vi "Begin.vi"() -> (0 "error out":errorcluster, 1 "CameraDevRef":T1)   [LabVIEW 2011]
doc: "Called before other user functions, this VI is expected to open initial I/O refnums, load in file data, and do all program initialization. Notice that the <B>error out</B> terminal is simply used for data flow. Wiring it to other structures or subVIs ensures that this VI runs first."
uses:
  Robot Global Data.vi
  <vilib>/Rock Robotics/WPI/MotorControl/WPI_MotorControlOpen Victor.vi
  <vilib>/Rock Robotics/SystemInterfaces/DIO/FPGA_DIOPWMChannel.ctl
  <vilib>/Rock Robotics/WPI/Joystick/WPI_JoystickDeviceEnum.ctl
  <vilib>/Rock Robotics/SystemInterfaces/DIO/FPGA_DIORelayChannel.ctl
  <vilib>/Rock Robotics/WPI/Relay/WPI_RelayDirection.ctl
  <vilib>/Rock Robotics/SystemInterfaces/Typedef/FPGA_TypedefDigitalModule.ctl
  <vilib>/Rock Robotics/SystemInterfaces/AI/FPGA_AIChannel.ctl
  <vilib>/Rock Robotics/WPI/Counter/WPI_CounterDigitalInputToDigitalSource.vi
  <vilib>/Rock Robotics/SystemInterfaces/DIO/FPGA_DIOChannel.ctl
  <vilib>/Rock Robotics/WPI/Encoder/WPI_EncoderType.ctl
  <vilib>/Rock Robotics/SystemInterfaces/AI/FPGA_AIGyroChannel.ctl
  <vilib>/Rock Robotics/WPI/MotorControl/WPI_MotorControlOpen Jaguar.vi
  <vilib>/Utility/file.llb/Read From Spreadsheet File (DBL).vi
  <vilib>/Rock Robotics/WPI/Camera/WPI_CameraDevRef.ctl
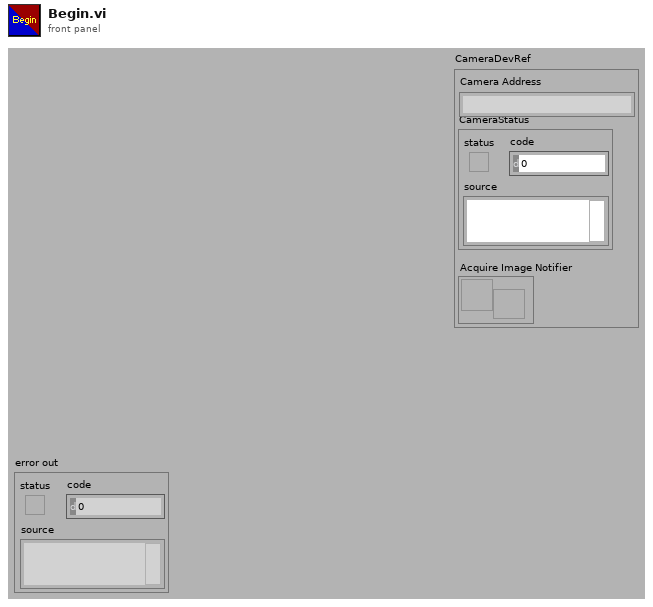
[diagram p1: front panel]
types:
  T1 = typedef "WPI_CameraDevRef.ctl" = cluster{"Camera Address":string, "CameraStatus":errorcluster, "Acquire Image Notifier":refnum<notifier>}
  T2 = typedef "FPGA_TypedefDigitalModule.ctl" = enum16{"Digital Module 1", "Digital Module 2"}
  T3 = typedef "FPGA_DIOPWMChannel.ctl" = enum8{"PWM 1", "PWM 2", "PWM 3", "PWM 4", "PWM 5", "PWM 6", "PWM 7", "PWM 8", "PWM 9", "PWM 10", "Invalid"}
  T4 = typedef "FPGA_AIGyroChannel.ctl" = enum8{"AI 1", "AI 2", "Invalid"}
  T5 = typedef "WPI_EncoderType.ctl" = enum16{"1x", "2x", "4x"}
  T6 = typedef "FPGA_DIOChannel.ctl" = enum8{"DIO 1", "DIO 2", "DIO 3", "DIO 4", "DIO 5", "DIO 6", "DIO 7", "DIO 8", "DIO 9", "DIO 10", "DIO 11", "DIO 12", "DIO 13", "DIO 14", "Invalid"}
  T7 = typedef "FPGA_AIChannel.ctl" = enum8{"AI 1", "AI 2", "AI 3", "AI 4", "AI 5", "AI 6", "AI 7", "AI 8", "Invalid"}
  T8 = typedef "FPGA_DIORelayChannel.ctl" = enum8{"Relay 1", "Relay 2", "Relay 3", "Relay 4", "Relay 5", "Relay 6", "Relay 7", "Relay 8", "Invalid"}
  T9 = typedef "WPI_RelayDirection.ctl" = enum16{"Both directions", "Forward only", "Reverse only"}
  T10 = typedef "WPI_JoystickDeviceEnum.ctl" = enum16{"USB 1", "USB 2", "USB 3", "USB 4", "Kinect 1", "Kinect 2"}
  T11 = typedef "WPI_CameraImageSize.ctl" = enum16{"640x480", "320x240", "160x120"}
  T12 = cluster{"fps":i32, "compression":i32, "Image Size":T11}
  T13 = typedef "WPI_I2CDevRef.ctl" = cluster{"DevStatus":errorcluster, "Digital Module":T2, "Device Address":u8}
  T14 = typedef "WPI_DigitalInputDevRef.ctl" = cluster{"DevStatus":errorcluster, "DIO Channel":T6, "Digital Module":T2}
  T15 = typedef "FPGA_CounterEncoderSourceConvertionLVSourceType.ctl" = cluster{"DevStatus":errorcluster, "AnalogTriggerMode?":bool, "DigitalMode":cluster{"Digital Module":T2, "DIO Channel":T16}, "AnalogTriggerMode":cluster{"AnalogTriggerIndex":T17, "OutputType":T18}}
  T16 = typedef "FPGA_DIODigitalSourceChannel.ctl" = enum8{"DIO 1", "DIO 2", "DIO 3", "DIO 4", "DIO 5", "DIO 6", "DIO 7", "DIO 8", "DIO 9", "DIO 10", "DIO 11", "DIO 12", "DIO 13", "DIO 14", "Disabled"}
  T17 = typedef "FPGA_AnalogTriggerIndex.ctl" = enum8{"Trig 0", "Trig 1", "Trig 2", "Trig 3", "Trig 4", "Trig 5", "Trig 6", "Trig 7", "Invalid"}
  T18 = typedef "FPGA_AnalogTriggerOutType.ctl" = enum16{"InWindow", "TriggerState", "Rising", "Falling"}
  T19 = typedef "WPI_MotorControlDeviceRef.ctl" = cluster{"DeviceStatus":errorcluster, "Type":enum16{"PWM", "CAN"}, "PWM":cluster{"Digital Module":T2, "PWM Channel":T3, "DeadBand":T20}, "CAN":cluster{"Device Number":u8, "Control Mode":T21, "Semaphore":T22, "Max Vout":dbl}, "Invert":bool, "TransformRef":T23, "InvTransformRef":T23}
  T20 = typedef "WPI_PWMDeadband.ctl" = cluster{"Name":string, "maxPositivePwm":i32, "minPositivePwm":i32, "centerPwm":i32, "maxNegativePwm":i32, "minNegativePwm":i32, "angularRange":u16}
  T21 = typedef "WPI_CANJaguar_ControlMode.ctl" = enum8{"Percent VBus", "Current", "Speed", "Position", "Voltage"}
  T22 = typedef "Semaphore RefNum" = refnum<k1>
  T23 = typedef "WPI_PWMTransform_ConPane.ctl" = refnum<vi>
  T24 = typedef "WPI_EncoderDevRef.ctl" = cluster{"DevStatus":errorcluster, "EncoderIndex":T25, "CounterIndex":T26, "DistancePerCount":dbl, "Decoding Type":T5}
  T25 = typedef "FPGA_EncoderIdx.ctl" = enum8{"Enc 0", "Enc 1", "Enc 2", "Enc 3", "Invalid"}
  T26 = typedef "FPGA_CounterCtrSystemIndex.ctl" = enum8{"Ctr 0", "Ctr 1", "Ctr 2", "Ctr 3", "Ctr 4", "Ctr 5", "Ctr 6", "Ctr 7", "Invalid"}
  T27 = typedef "WPI_CameraWhite Balance Values.ctl" = enum16{"Auto", "Fixed indoor", "Fixed outdoor 1", "Fixed outdoor 2", "Fixed fluorescent 1", "Fixed fluorescent 2", "Hold current"}
  T28 = typedef "WPI_CameraExposure Values.ctl" = enum16{"Auto", "Flicker-free 50 Hz", "Flicker-free 60 Hz", "Hold current"}
  T29 = typedef "WPI_ServoDeviceRef.ctl" = cluster{"DeviceStatus":errorcluster, "Digital Module":T2, "PWM Channel":T3, "DeadBand":T20}
  T30 = typedef "WPI_AnalogChannelDevRef.ctl" = cluster{"DevStatus":errorcluster, "Analog Module":T31, "Analog Channel":T7}
  T31 = typedef "FPGA_TypedefAnalogModule.ctl" = enum16{"Analog Module 1", "Analog Module 2"}
  T32 = typedef "WPI_JoystickDevRef.ctl" = cluster{"Device":T10}
  T33 = typedef "WPI_GyroDevRef.ctl" = cluster{"DevStatus":errorcluster, "Analog Module":T31, "Analog Channel":T7, "Offset":dbl, "Gain (VoltsPerDegree/Second)":dbl}
  T34 = typedef "WPI_RelayDevRef.ctl" = cluster{"DevStatus":errorcluster, "Relay Channel":T8, "Digital Module":T2, "Relay Direction":T9}
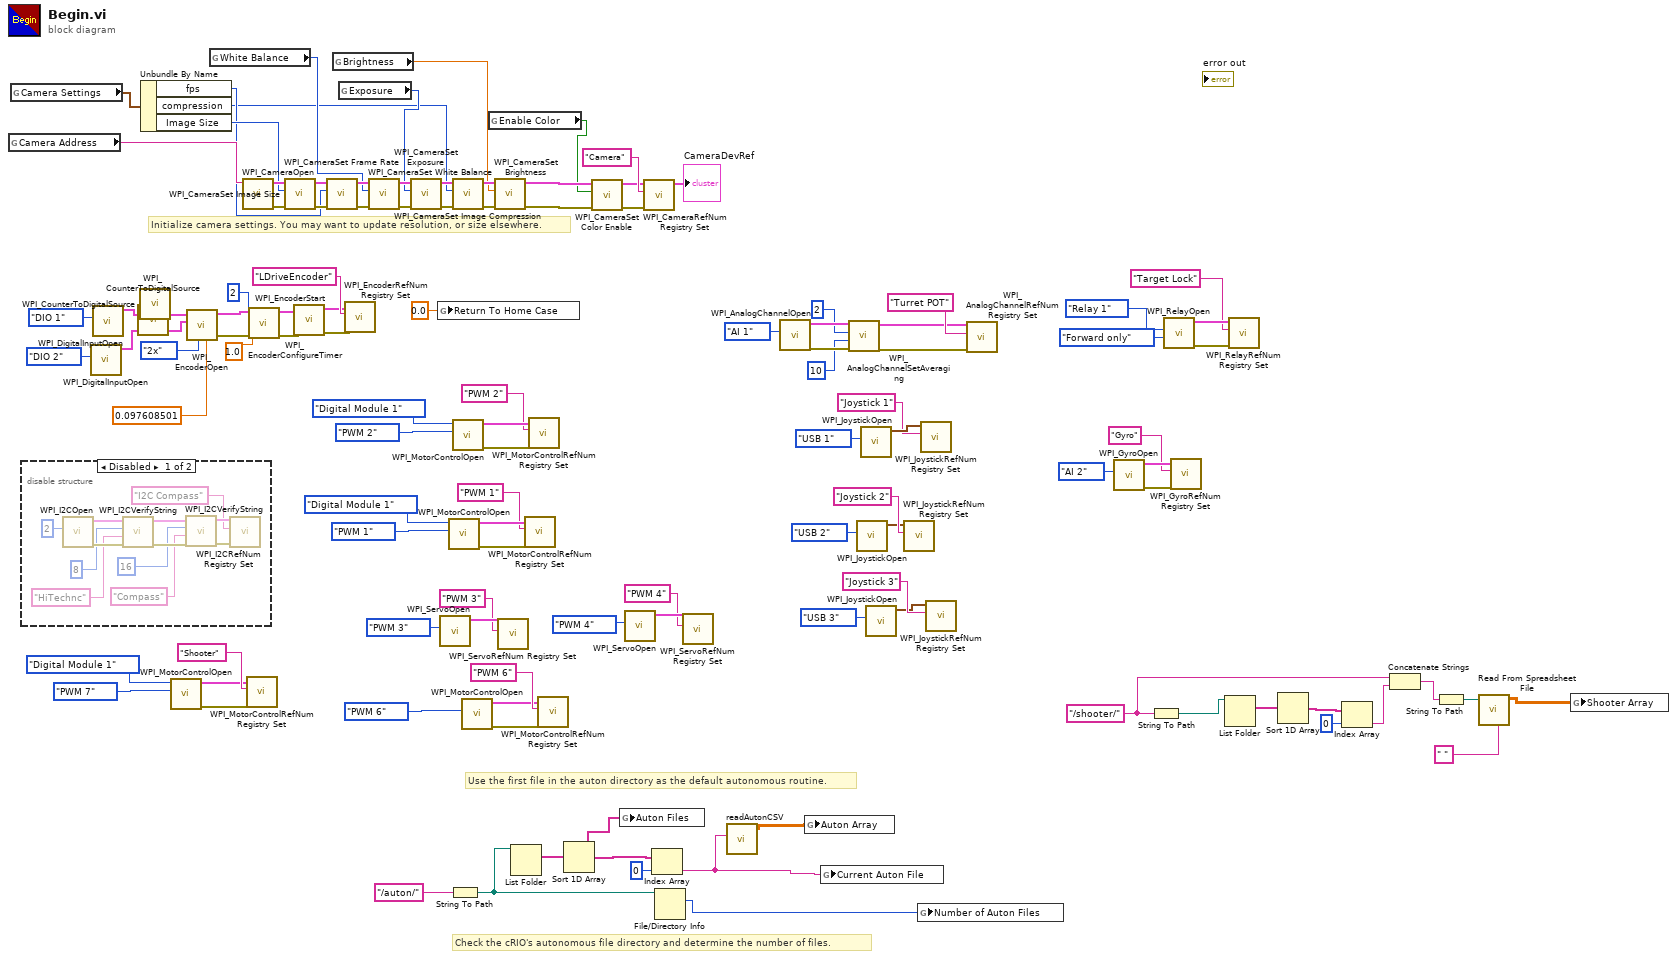
[diagram p0: block diagram]
diagram:
  w11 = "/shooter/" ("string")
  # "Check the cRIO's autonomous file directory and determine the number of files."
  # "Use the first file in the auton directory as the default autonomous routine."
  # "Initialize camera settings. You may want to update resolution, or size elsewhere."
  n1 = global read "Robot Global Data.vi" "Camera Address"() -> (w101:string)
  n2 = global read "Robot Global Data.vi" "Camera Settings"() -> (w73:T12)
  n3 = disable-structure shown="Disabled" {
    frame Disabled {
      n4 = call <vilib>:"WPI_I2COpen.vi"("Device Address"=u8 2) -> ("error out"=w126:errorcluster, "I2CDevRef"=w125:T13)  [unwired: 9 in]
      n5 = call <vilib>:"WPI_I2CVerifyString.vi"("error in (no error)"=w126, "Expected"="HiTechnc", "Register Address"=u8 8, "I2CDevRef"=w125) -> ("error out"=w124:errorcluster, "I2CDevRef"=w123:T13)  [unwired: 6 in]
      n6 = call <vilib>:"WPI_I2CVerifyString.vi"("error in (no error)"=w124, "Expected"="Compass", "Register Address"=u8 16, "I2CDevRef"=w123) -> ("error out"=w122:errorcluster, "I2CDevRef"=w121:T13)  [unwired: 6 in]
      n7 = call <vilib>:"WPI_I2CRefNum Registry Set.vi"("error in (no error)"=w122, "refnum name"="I2C Compass", "I2CDevRef"=w121) -> ()  [unwired: 7 in, 2 out]
    }
    frame Enabled {
    }
  }
  n8 = call <vilib>:"WPI_DigitalInputOpen.vi"("DIO Channel"=FPGA_DIOChannel."DIO 2") -> ("DigitalInputDevRef"=w38:T14)  [unwired: 9 in, 1 out]
  n9 = call <vilib>:"WPI_DigitalInputOpen.vi"("DIO Channel"=FPGA_DIOChannel."DIO 1") -> ("DigitalInputDevRef"=w41:T14)  [unwired: 9 in, 1 out]
  n10 = call-poly <vilib>:"WPI_CounterToDigitalSource.vi"("DigitalInputDevRef"=w38) -> ("Digital Source"=w37:T15)  [unwired: 6 in]
  n11 = call-poly <vilib>:"WPI_CounterToDigitalSource.vi"("DigitalInputDevRef"=w41) -> ("Digital Source"=w42:T15)  [unwired: 6 in]
  n12 = Unbundle By Name(w73) -> ("fps"=w71:i32, "compression"=w68:i32, "Image Size"=w72:T11)
  n13 = call-poly <vilib>:"WPI_MotorControlOpen.vi"("PWM Channel"=FPGA_DIOPWMChannel."PWM 7", "Digital Module (Module 1)"=FPGA_TypedefDigitalModule."Digital Module 1") -> ("error out"=w20:errorcluster, "MotorControlDeviceRef"=w18:T19)  [unwired: 8 in]
  n14 = call <vilib>:"WPI_EncoderOpen.vi"("DistancePerCount"=0.097608501, "Decoding Type"=WPI_EncoderType."2x", "BSource"=w37, "ASource"=w42) -> ("error out"=w33:errorcluster, "EncoderDevRef"=w32:T24)  [unwired: 6 in]
  n15 = global read "Robot Global Data.vi" "White Balance"() -> (w70:T27)
  n16 = call <vilib>:"WPI_CameraOpen.vi"("Camera Address"=w101) -> ("error out"=w107:errorcluster, "CameraDevRef"=w108:T1)  [unwired: 1 in, 8 out]
  n17 = call <vilib>:"WPI_MotorControlRefNum Registry Set.vi"("error in (no error)"=w20, "refnum name"="Shooter", "MotorControlDevRef"=w18) -> ()  [unwired: 7 in, 2 out]
  n18 = call <vilib>:"WPI_EncoderConfigureTimer.vi"("error in (no error)"=w33, "Number Samples to Average"=u8 2, "Minimum Rate"=1.0, "EncoderDevRef"=w32) -> ("error out"=w28:errorcluster, "EncoderDevRef"=w29:T24)  [unwired: 6 in]
  n19 = call <vilib>:"WPI_CameraSet Image Size.vi"("error in (no error)"=w107, "Image Size"=w72, "CameraDevRef"=w108) -> ("error out"=w106:errorcluster, "CameraDevRef Out"=w109:T1)  [unwired: 7 out]
  n20 = call <vilib>:"WPI_EncoderStart.vi"("error in (no error)"=w28, "EncoderDevRef"=w29) -> ("error out"=w26:errorcluster, "EncoderDevRef"=w27:T24)  [unwired: 8 in]
  n21 = call <vilib>:"WPI_CameraSet Frame Rate.vi"("error in (no error)"=w106, "Frame Rate (fps)"=w71, "CameraDevRef"=w109) -> ("error out"=w105:errorcluster, "CameraDevRef Out"=w111:T1)  [unwired: 7 out]
  n22 = global read "Robot Global Data.vi" "Brightness"() -> (w67:dbl)
  n23 = global read "Robot Global Data.vi" "Exposure"() -> (w69:T28)
  n24 = call <vilib>:"WPI_EncoderRefNum Registry Set.vi"("error in (no error)"=w26, "refnum name"="LDriveEncoder", "EncoderDevRef"=w27) -> ()  [unwired: 7 in, 2 out]
  n25 = call <vilib>:"WPI_CameraSet White Balance.vi"("error in (no error)"=w105, "White Balance"=w70, "CameraDevRef"=w111) -> ("error out"=w104:errorcluster, "CameraDevRef Out"=w110:T1)  [unwired: 7 out]
  n26 = call <vilib>:"WPI_CameraSet Exposure.vi"("error in (no error)"=w104, "Exposure"=w69, "CameraDevRef"=w110) -> ("error out"=w103:errorcluster, "CameraDevRef Out"=w113:T1)  [unwired: 7 out]
  n27 = global write "Robot Global Data.vi" "Return To Home Case"(0.0 ("Return To Home Case")) -> ()
  n28 = call <vilib>:"WPI_ServoOpen.vi"("PWM Channel"=FPGA_DIOPWMChannel."PWM 3") -> ("ServoDeviceRef"=w87:T29)  [unwired: 9 in, 1 out]
  n29 = call-poly <vilib>:"WPI_MotorControlOpen.vi"("PWM Channel"=FPGA_DIOPWMChannel."PWM 1", "Digital Module (Module 1)"=FPGA_TypedefDigitalModule."Digital Module 1") -> ("error out"=w93:errorcluster, "MotorControlDeviceRef"=w96:T19)  [unwired: 8 in]
  n30 = String To Path(string="/auton/") -> (path=w49:path)
  n31 = call <vilib>:"WPI_CameraSet Image Compression.vi"("error in (no error)"=w103, "Compression"=w68, "CameraDevRef"=w113) -> ("error out"=w102:errorcluster, "CameraDevRef Out"=w112:T1)  [unwired: 7 out]
  n32 = call-poly <vilib>:"WPI_MotorControlOpen.vi"("PWM Channel"=FPGA_DIOPWMChannel."PWM 2", "Digital Module (Module 1)"=FPGA_TypedefDigitalModule."Digital Module 1") -> ("error out"=w94:errorcluster, "MotorControlDeviceRef"=w99:T19)  [unwired: 8 in]
  n33 = call-poly <vilib>:"WPI_MotorControlOpen.vi"("PWM Channel"=FPGA_DIOPWMChannel."PWM 6") -> ("error out"=w82:errorcluster, "MotorControlDeviceRef"=w80:T19)  [unwired: 9 in]
  n34 = global read "Robot Global Data.vi" "Enable Color"() -> (w62:bool)
  n35 = call <vilib>:"WPI_CameraSet Brightness.vi"("error in (no error)"=w102, "Brightness"=w67, "CameraDevRef"=w112) -> ("error out"=w65:errorcluster, "CameraDevRef Out"=w66:T1)  [unwired: 7 out]
  n36 = call <vilib>:"WPI_ServoRefNum Registry Set.vi"("refnum name"="PWM 3", "ServoDeviceRef"=w87) -> ()  [unwired: 8 in, 2 out]
  n37 = List Folder(path=w49) -> (filenames=w48:string[])  [unwired: 1 in, 5 out]
  n38 = call <vilib>:"WPI_MotorControlRefNum Registry Set.vi"("error in (no error)"=w93, "refnum name"="PWM 1", "MotorControlDevRef"=w96) -> ()  [unwired: 7 in, 2 out]
  n39 = call <vilib>:"WPI_MotorControlRefNum Registry Set.vi"("error in (no error)"=w94, "refnum name"="PWM 2", "MotorControlDevRef"=w99) -> ()  [unwired: 7 in, 2 out]
  n40 = call <vilib>:"WPI_MotorControlRefNum Registry Set.vi"("error in (no error)"=w82, "refnum name"="PWM 6", "MotorControlDevRef"=w80) -> ()  [unwired: 7 in, 2 out]
  n41 = Sort 1D Array(array=w48) -> (sorted array=w43:string[])
  n42 = call <vilib>:"WPI_CameraSet Color Enable.vi"("error in (no error)"=w65, "Color Enabled"=w62, "CameraDevRef"=w66) -> ("error out"=w63:errorcluster, "CameraDevRef Out"=w64:T1)  [unwired: 7 in]
  n43 = global write "Robot Global Data.vi" "Auton Files"(w43) -> ()
  n44 = call <vilib>:"WPI_ServoOpen.vi"("PWM Channel"=FPGA_DIOPWMChannel."PWM 4") -> ("ServoDeviceRef"=w85:T29)  [unwired: 9 in, 1 out]
  n45 = call <vilib>:"WPI_CameraRefNum Registry Set.vi"("error in (no error)"=w63, "refnum name"="Camera", "CameraDevRef"=w64) -> ("CameraDevRef"=→"CameraDevRef":T1)  [unwired: 8 out]
  n46 = Index Array(array=w43, index=0) -> (element=w45:string)
  n47 = File/Directory Info(path=w49) -> (size=w46:i64)  [unwired: 1 in, 6 out]
  n48 = call <vilib>:"WPI_ServoRefNum Registry Set.vi"("refnum name"="PWM 4", "ServoDeviceRef"=w85) -> ()  [unwired: 8 in, 2 out]
  n49 = call "readAutonCSV.vi"("AutonFile"=w45) -> ("AutonArray"=w44:dbl[][])  [unwired: 7 in]
  n50 = call <vilib>:"WPI_AnalogChannelOpen.vi"("Analog Channel"=FPGA_AIChannel."AI 1") -> ("error out"=w3:errorcluster, "AIDeviceRef"=w6:T30)  [unwired: 9 in]
  n51 = global write "Robot Global Data.vi" "Auton Array"(w44) -> ()
  n52 = global write "Robot Global Data.vi" "Current Auton File"(w45) -> ()
  n53 = call <vilib>:"WPI_AnalogChannelSetAveraging.vi"("error in (no error)"=w3, "OversampleBits"=u8 10, "AverageBits"=u8 2, "AIDeviceRef"=w6) -> ("error out"=w4:errorcluster, "AIDeviceRef"=w5:T30)  [unwired: 6 in]
  n54 = call <vilib>:"WPI_JoystickOpen.vi"("JoystickDevice"=WPI_JoystickDeviceEnum."USB 2") -> ("JoystickDevRef"=w89:T32)  [unwired: 10 in]
  n55 = call <vilib>:"WPI_JoystickOpen.vi"("JoystickDevice"=WPI_JoystickDeviceEnum."USB 1") -> ("JoystickDevRef"=w92:T32)  [unwired: 10 in]
  n56 = call <vilib>:"WPI_JoystickOpen.vi"("JoystickDevice"=WPI_JoystickDeviceEnum."USB 3") -> ("JoystickDevRef"=w77:T32)  [unwired: 10 in]
  n57 = call <vilib>:"WPI_JoystickRefNum Registry Set.vi"("refnum name"="Joystick 2", "JoystickDevRef"=w89) -> ()  [unwired: 8 in, 2 out]
  n58 = global write "Robot Global Data.vi" "Number of Auton Files"(w46) -> ()
  n59 = call <vilib>:"WPI_JoystickRefNum Registry Set.vi"("refnum name"="Joystick 1", "JoystickDevRef"=w92) -> ()  [unwired: 8 in, 2 out]
  n60 = call <vilib>:"WPI_JoystickRefNum Registry Set.vi"("refnum name"="Joystick 3", "JoystickDevRef"=w77) -> ()  [unwired: 8 in, 2 out]
  n61 = call <vilib>:"WPI_AnalogChannelRefNum Registry Set.vi"("error in (no error)"=w4, "refnum name"="Turret POT", "AIDeviceRef"=w5) -> ()  [unwired: 7 in, 2 out]
  n62 = call <vilib>:"WPI_GyroOpen.vi"("Analog Channel"=FPGA_AIGyroChannel."AI 2") -> ("error out"=w25:errorcluster, "GyroDevRef"=w24:T33)  [unwired: 8 in, 1 out]
  n63 = String To Path(string=w11) -> (path=w13:path)
  n64 = call <vilib>:"WPI_RelayOpen.vi"("Relay Direction"=WPI_RelayDirection."Forward only", "Relay Channel"=FPGA_DIORelayChannel."Relay 1") -> ("error out"=w59:errorcluster, "RelayDevRef"=w60:T34)  [unwired: 8 in]
  n65 = call <vilib>:"WPI_GyroRefNum Registry Set.vi"("error in (no error)"=w25, "refnum name"="Gyro", "GyroDevRef"=w24) -> ()  [unwired: 7 in, 2 out]
  n66 = List Folder(path=w13) -> (filenames=w12:string[])  [unwired: 1 in, 5 out]
  n67 = call <vilib>:"WPI_RelayRefNum Registry Set.vi"("error in (no error)"=w59, "refnum name"="Target Lock", "RelayDevRef"=w60) -> ()  [unwired: 7 in, 2 out]
  n68 = Sort 1D Array(array=w12) -> (sorted array=w15:string[])
  n69 = Index Array(array=w15, index=0) -> (element=w10:string)
  n70 = Concatenate Strings(w11, w10) -> (w9:string)
  n71 = String To Path(string=w9) -> (path=w8:path)
  n72 = call-poly <vilib>:"Read From Spreadsheet File.vi"("delimiter (\\t)"=" " ("delimiter (\\t)"), "file path (dialog if empty)"=w8) -> ("all rows"=w7:dbl[][])  [unwired: 5 in, 4 out]
  n73 = global write "Robot Global Data.vi" "Shooter Array"(w7) -> ()
